vi "Global 1.vi"() -> ()   [LabVIEW 2018]
panel:
  out "Numeric":i16
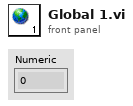
[diagram p1: front panel]
diagram:
